vi "FTW-Benchmark-JSON-DeserializeXNode.vi"() -> ()   [LabVIEW 2013]
uses:
  source/JSON/FTW-JSON-Core-LibraryFilepath.vi
  source/Reflection/FTW-Reflection-Type.vi
  source/JSON/FTW-JSON-Core-GetFlattenedValue.vi
  source/JSON/FTW-JSON-Core-LibraryError.vi
  source/CodeGen/JSON Deserialize/FTW-JSON-Deserialize.xnode
  source/JSON/FTW-JSON-Native-GetFlattenedValue.vi
  source/JSON/FTW-JSON-Validate.vi
panel:
  out "Average Iteration Time":dbl format="%.3psec"
  out "Test Time":dbl format="%<%H:%M:%S%3u>t"
  in  "Parallel Instances":i32=64
  in  "Iterations":i32=1000
  out "Pass":bool
  out "error out":errorcluster
  out "element":T1 {"subobject"."EXT" format="%_32g"; "subobject"."DBL" format="%_32g"; "subobject"."SGL" format="%_32g"; "EXT" format="%_32g"; "DBL" format="%_32g"; "SGL" format="%_32g"}
  in  "Object":string="{\n  \"booleanfalse\": false,\n  \"booleantrue\": true,\n  \"U8\": 8,\n  \"U16\": 16,\n  \"U32\": 32,\n  \"U64\": 64,\n  \"I8\": -8,\n  \"I16\": -16,\n  \"I32\": -32,\n  \"I64\": -64,\n  \"SGL\": 1.23456789,\n  \"DBL\": 1.2345678901234567,\n  \"EXT\": 1.2345678901234567,\n  \"nullstring\": null,\n  \"stringempty\": \"\",\n  \"stringHW\": \"Hello World\",\n  \"EnumU8\": \"U8\",\n  \"EnumU16\": \"U16\",\n  \"EnumU32\": \"U32\",\n  \"Path\": \"c:\\\\some folder\\\\some file.txt\",\n  \"array\": [1,2,3],\n  \"visa resource\": \"myresource\",\n  \"VIrefnum\": \"0x123456789ABCDEF0\",\n  \"subobject\": {\n    \"booleanfalse\": false,\n    \"booleantrue\": true,\n    \"U8\": 8,\n    \"U16\": 16,\n    \"U32\": 32,\n    \"U64\": 64,\n    \"I8\": -8,\n    \"I16\": -16,\n    \"I32\": -32,\n    \"I64\": -64,\n    \"SGL\": 1.23456789,\n    \"DBL\": 1.2345678901234567,\n    \"EXT\": 1.2345678901234567,\n    \"nullstring\": null,\n    \"stringempty\": \"\",\n    \"stringHW\": \"Hello World\",\n    \"EnumU8\": \"U8\",\n    \"EnumU16\": \"U16\",\n    \"EnumU32\": \"U32\",\n    \"Path\": \"c:\\\\some folder\\\\some file.txt\",\n    \"array\": [4,5,6],\n    \"visa resource\": \"myresource\",\n    \"VIrefnum\": \"0x123456789ABCDEF0\"\n  },\n  \"unusedpair\": \"whatever\"\n}"
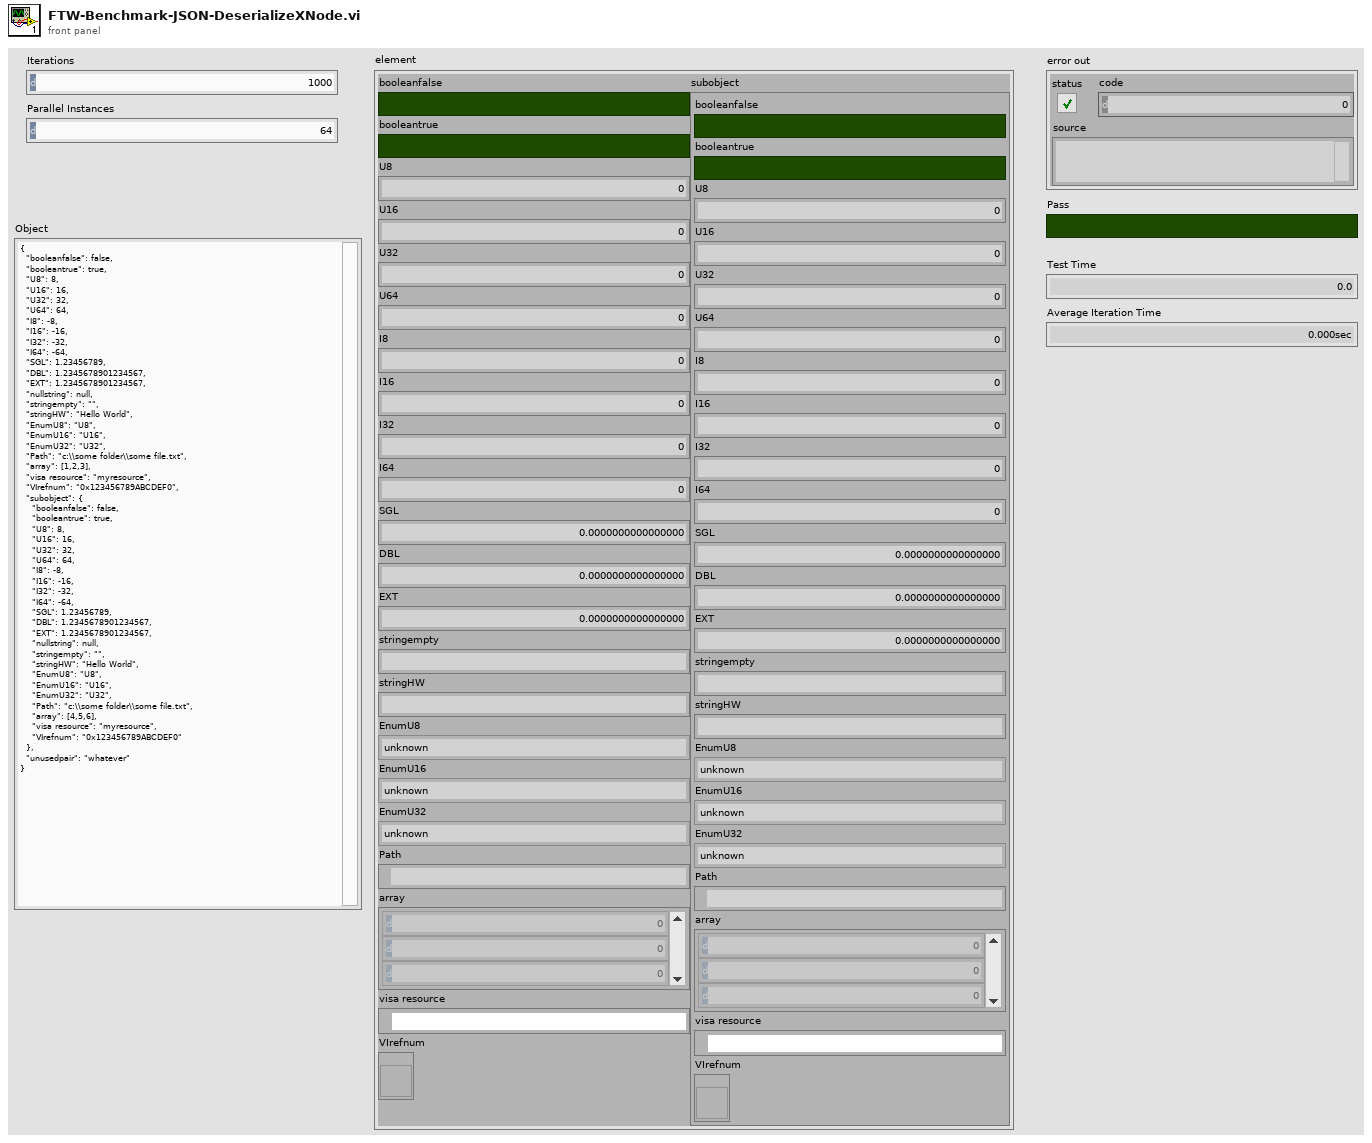
[diagram p1: front panel]
types:
  T1 = cluster{"booleanfalse":bool, "booleantrue":bool, "U8":u8, "U16":u16, "U32":u32, "U64":u64, "I8":i8, "I16":i16, "I32":i32, "I64":i64, "SGL":sgl, "DBL":dbl, "EXT":ext, "stringempty":string, "stringHW":string, "EnumU8":enum8{"unknown", "U8"}, "EnumU16":enum16{"unknown", "U16"}, "EnumU32":enum32{"unknown", "U32"}, "Path":path, "array":i32[], "visa resource":refnum<visa-resource-name>, "VIrefnum":refnum<vi>, "subobject":cluster{"booleanfalse":bool, "booleantrue":bool, "U8":u8, "U16":u16, "U32":u32, "U64":u64, "I8":i8, "I16":i16, "I32":i32, "I64":i64, "SGL":sgl, "DBL":dbl, "EXT":ext, "stringempty":string, "stringHW":string, "EnumU8":enum8{"unknown", "U8"}, "EnumU16":enum16{"unknown", "U16"}, "EnumU32":enum32{"unknown", "U32"}, "Path":path, "array":i32[], "visa resource":refnum<visa-resource-name>, "VIrefnum":refnum<vi>}}
  T2 = cluster{"booleanfalse":bool, "booleantrue":bool, "U8":u8, "U16":u16, "U32":u32, "U64":u64, "I8":i8, "I16":i16, "I32":i32, "I64":i64, "SGL":sgl, "DBL":dbl, "EXT":ext, "stringempty":string, "stringHW":string, "EnumU8":enum8{"unknown", "U8"}, "EnumU16":enum16{"unknown", "U16"}, "EnumU32":enum32{"unknown", "U32"}, "Path":path, "array":i32[], "visa resource":refnum<visa-resource-name>, "VIrefnum":refnum<vi>}
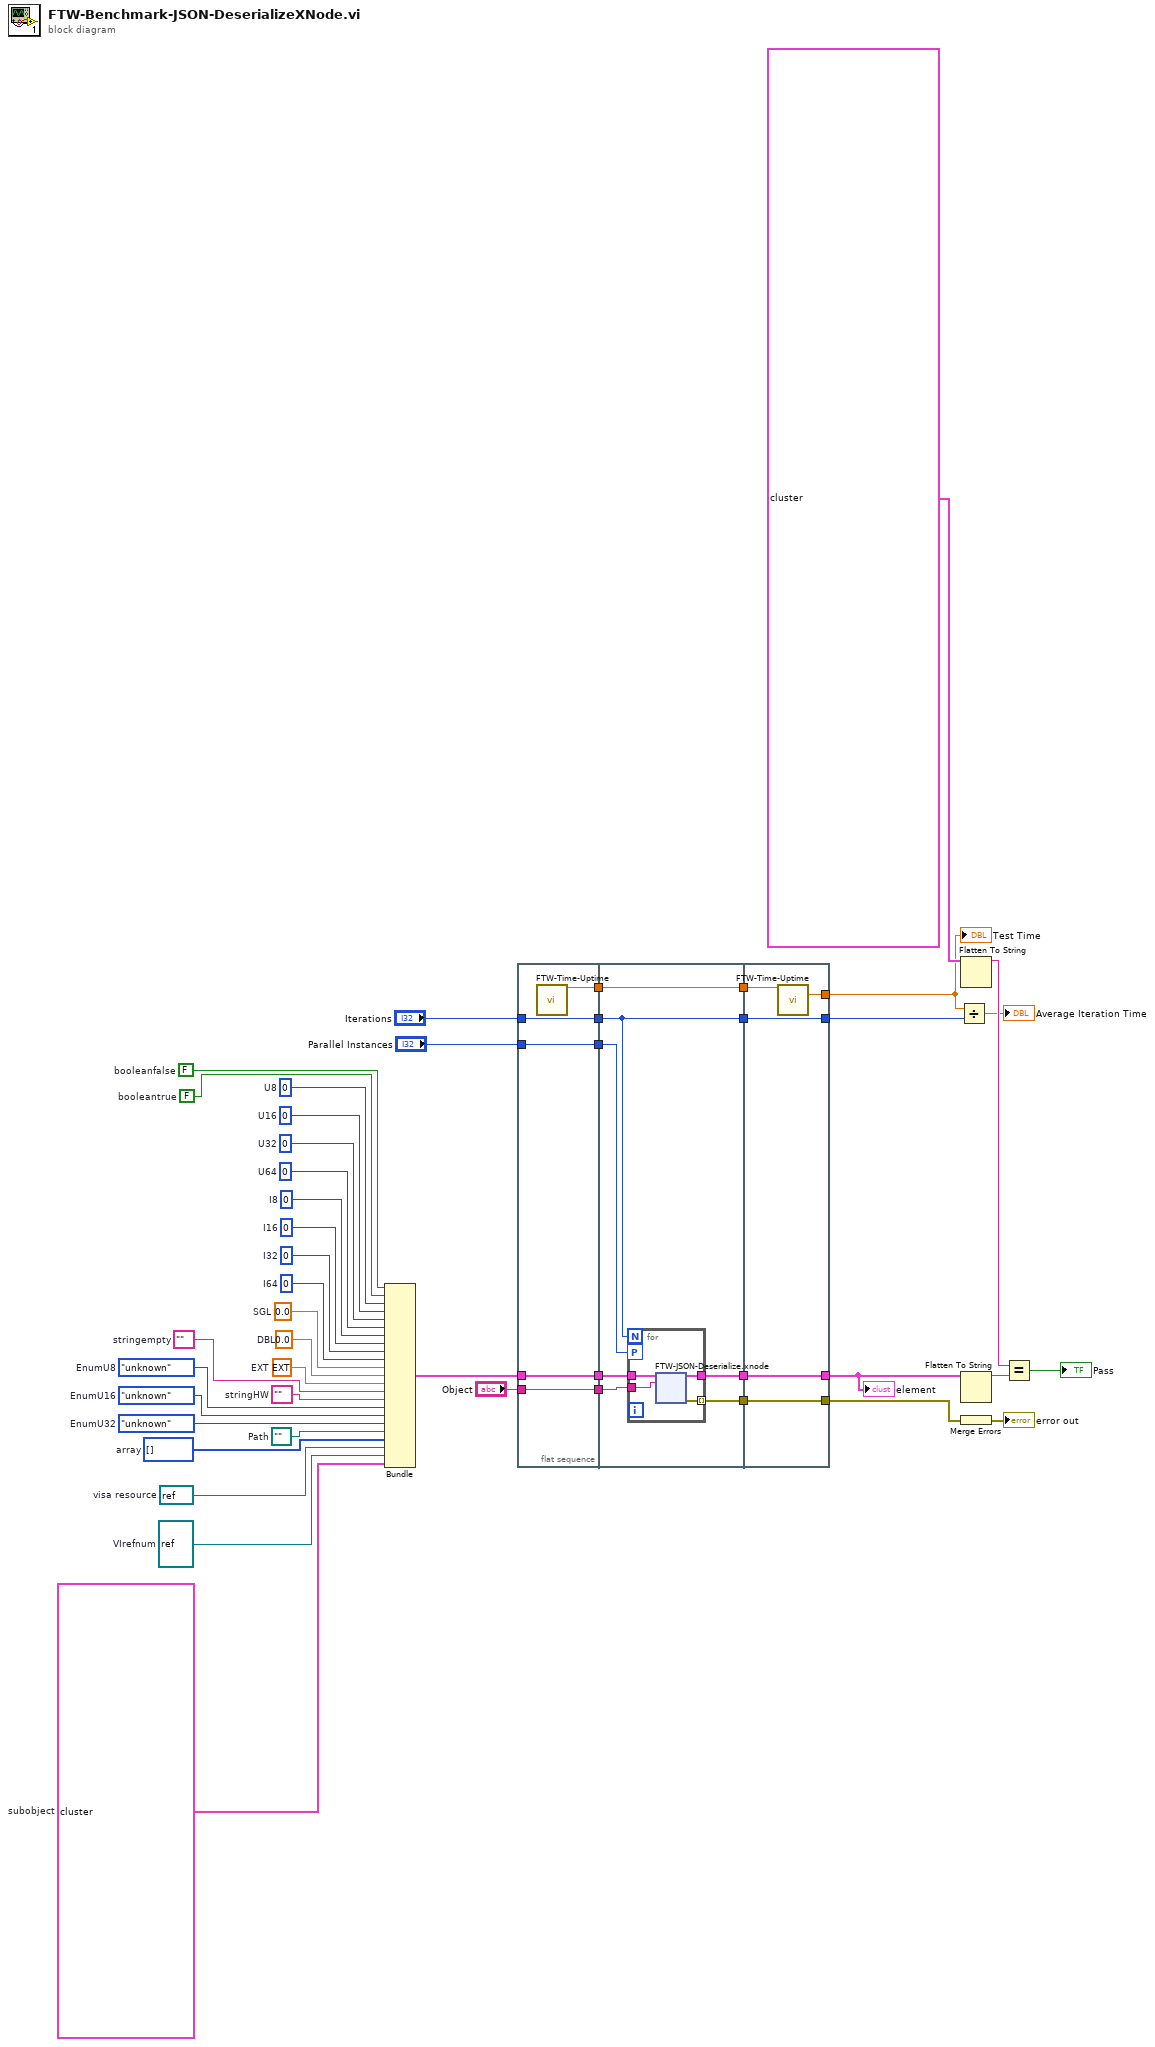
[diagram p0: block diagram]
diagram:
  w16 = refnum<vi> refnum  # VIrefnum
  w22 = refnum<visa-resource-name> refnum  # visa resource
  w23 = i32[] []  # array
  w24 = path ""  # Path
  w25 = T2 {"booleanfalse"=FALSE, "booleantrue"=FALSE, "U8"=0, "U16"=0, "U32"=0, "U64"=0, "I8"=0, "I16"=0, "I32"=0, "I64"=0, "SGL"=0.0, "DBL"=0.0, "EXT"=0.0, "stringempty"="", "stringHW"="", "EnumU8"=enum."unknown", "EnumU16"=enum."unknown", "EnumU32"=enum."unknown", "Path"=path "", "array"=[], "visa resource"="", "VIrefnum"=refnum}  # subobject
  w26 = enum32{"unknown", "U32"}."unknown"  # EnumU32
  w27 = enum16{"unknown", "U16"}."unknown"  # EnumU16
  w28 = enum8{"unknown", "U8"}."unknown"  # EnumU8
  w29 = ""  # stringHW
  w30 = ""  # stringempty
  w32 = FALSE  # booleantrue
  w33 = FALSE  # booleanfalse
  w34 = ext 0.0  # EXT
  w35 = 0.0  # DBL
  w36 = sgl 0.0  # SGL
  w37 = i64 0  # I64
  w38 = 0  # I32
  w39 = i16 0  # I16
  w40 = i8 0  # I8
  w41 = u64 0  # U64
  w42 = u32 0  # U32
  w43 = u16 0  # U16
  w44 = u8 0  # U8
  n1 = Bundle("booleanfalse"=w33, "booleantrue"=w32, "U8"=w44, "U16"=w43, "U32"=w42, "U64"=w41, "I8"=w40, "I16"=w39, "I32"=w38, "I64"=w37, "SGL"=w36, "DBL"=w35, "EXT"=w34, "stringempty"=w30, "stringHW"=w29, "EnumU8"=w28, "EnumU16"=w27, "EnumU32"=w26, "Path"=w24, "array"=w23, "visa resource"=w22, "VIrefnum"=w16, "subobject"=w25) -> (w31:T1)  [unwired: 1 in]
  n2 = flat-sequence {
    tunnel: w31 -> [w50]
    tunnel: "Object" -> [w51]
    tunnel: [w51] -> w15
    tunnel: [w50] -> w14
    tunnel: "Iterations" -> [w49]
    tunnel: [w49] -> w10
    tunnel: "Parallel Instances" -> [w48]
    tunnel: [w48] -> w8
    tunnel: [w47] -> w5
    tunnel: w15 -> [w58]
    tunnel: w14 -> [w56]
    tunnel: [w57] -> w13
    tunnel: [w55] -> w12
    tunnel: w10 -> [w52]
    tunnel: w8 -> [w54]
    tunnel: [w53] -> w6
    tunnel: w5 -> [w53]
    tunnel: [w52] -> w4
    tunnel: [w117] -> w20
    tunnel: [w118] -> w45
    tunnel: w13 -> [w118]
    tunnel: w12 -> [w117]
    tunnel: w6 -> [w116]
    tunnel: [w115] -> w3
    tunnel: w4 -> [w114]
    tunnel: [w114] -> w2
    frame #0 {
      n3 = call "FTW-Time-Uptime.vi"() -> ("Current Uptime"=w47:dbl)  [unwired: 13 in, 2 out]
    }
    frame #1 {
      n4 = for {
        N: w52 -> [_]
        tunnel: w58 -> [w62]
        tunnel: [w61] -> w57 mode=indexing
        tunnel: w56 -> [w60]
        tunnel: [w59] -> w55
        workers-P: w54 -> [_]
        n5 = xnode "FTW-JSON-Deserialize.xnode"("Type and Defaults"=w60, "JSON String"=w62) -> ("Values"=w59:T1, "error out"=w61:errorcluster)  [unwired: 1 in]
      }
    }
    frame #2 {
      n6 = call "FTW-Time-Uptime.vi"("Previous Uptime"=w116) -> ("Elapsed Time"=w115:dbl)  [unwired: 12 in, 2 out]
    }
  }
  n7 = Divide(x=w3, y=w2) -> (x/y=→"Average Iteration Time":dbl)
  n8 = Flatten To String(anything=T1 {"booleanfalse"=FALSE, "booleantrue"=TRUE, "U8"=8, "U16"=16, "U32"=32, "U64"=64, "I8"=-8, "I16"=-16, "I32"=-32, "I64"=-64, "SGL"=1.2345679, "DBL"=1.2345678901234567, "EXT"=1.2345678901234567, "stringempty"="", "stringHW"="Hello World", "EnumU8"=enum."U8", "EnumU16"=enum."U16", "EnumU32"=enum."U32", "Path"=path "c:/some folder/some file.txt", "array"=[1, 2, 3], "visa resource"="myresource", "VIrefnum"=refnum, "subobject"={"booleanfalse"=FALSE, "booleantrue"=TRUE, "U8"=8, "U16"=16, "U32"=32, "U64"=64, "I8"=-8, "I16"=-16, "I32"=-32, "I64"=-64, "SGL"=1.2345679, "DBL"=1.2345678901234567, "EXT"=1.2345678901234567, "stringempty"="", "stringHW"="Hello World", "EnumU8"=enum."U8", "EnumU16"=enum."U16", "EnumU32"=enum."U32", "Path"=path "c:/some folder/some file.txt", "array"=[4, 5, 6], "visa resource"="myresource", "VIrefnum"=refnum}} ("element")) -> (data string=w21:string)  [unwired: 3 in, 2 out]
  n9 = Flatten To String(anything=w20) -> (data string=w19:string)  [unwired: 3 in, 2 out]
  n10 = Merge Errors(w45) -> (→"error out":errorcluster)
  n11 = Equal?(x=w21, y=w19) -> (x = y?=→"Pass":bool)
  "element" <- w20
  "Test Time" <- w3
